vi "Stitch bottom tier.vi"(4 "Bottom tier Stitched Image":T1(plugin-control), 6 "Initial frame":bool, 8 "error in (no error)":errorcluster, 10 "Ctrl refs":T2, 11 "Input stitched image":T1) -> (0 "error out":errorcluster, 3 "Stitched Image":T1(plugin-control))   [LabVIEW 2013]
uses:
  <vilib>/vision/Image Controls.llb/IMAQ Image.ctl
  Typedefs/8-bit video export window ctrl refs.ctl
  Patch-Vol video generator/Typedefs/Bright-Contr-Gamma cluster.ctl
  Typedefs/Speed graph behaviour enum.ctl
  <vilib>/vision/NI_Vision_Development_Module.lvlib
panel:
  in  "AVI File Path":path=path "F:/Recovered data 03-24-2015 at 11_16_03/NTFS 1/LostFiles1/TimeLapse 03_10_2014 17-26-28 zoom1_50ns_MF_export/Green Channel 1.avi"
  out "Input stitched image":T1(plugin-control)
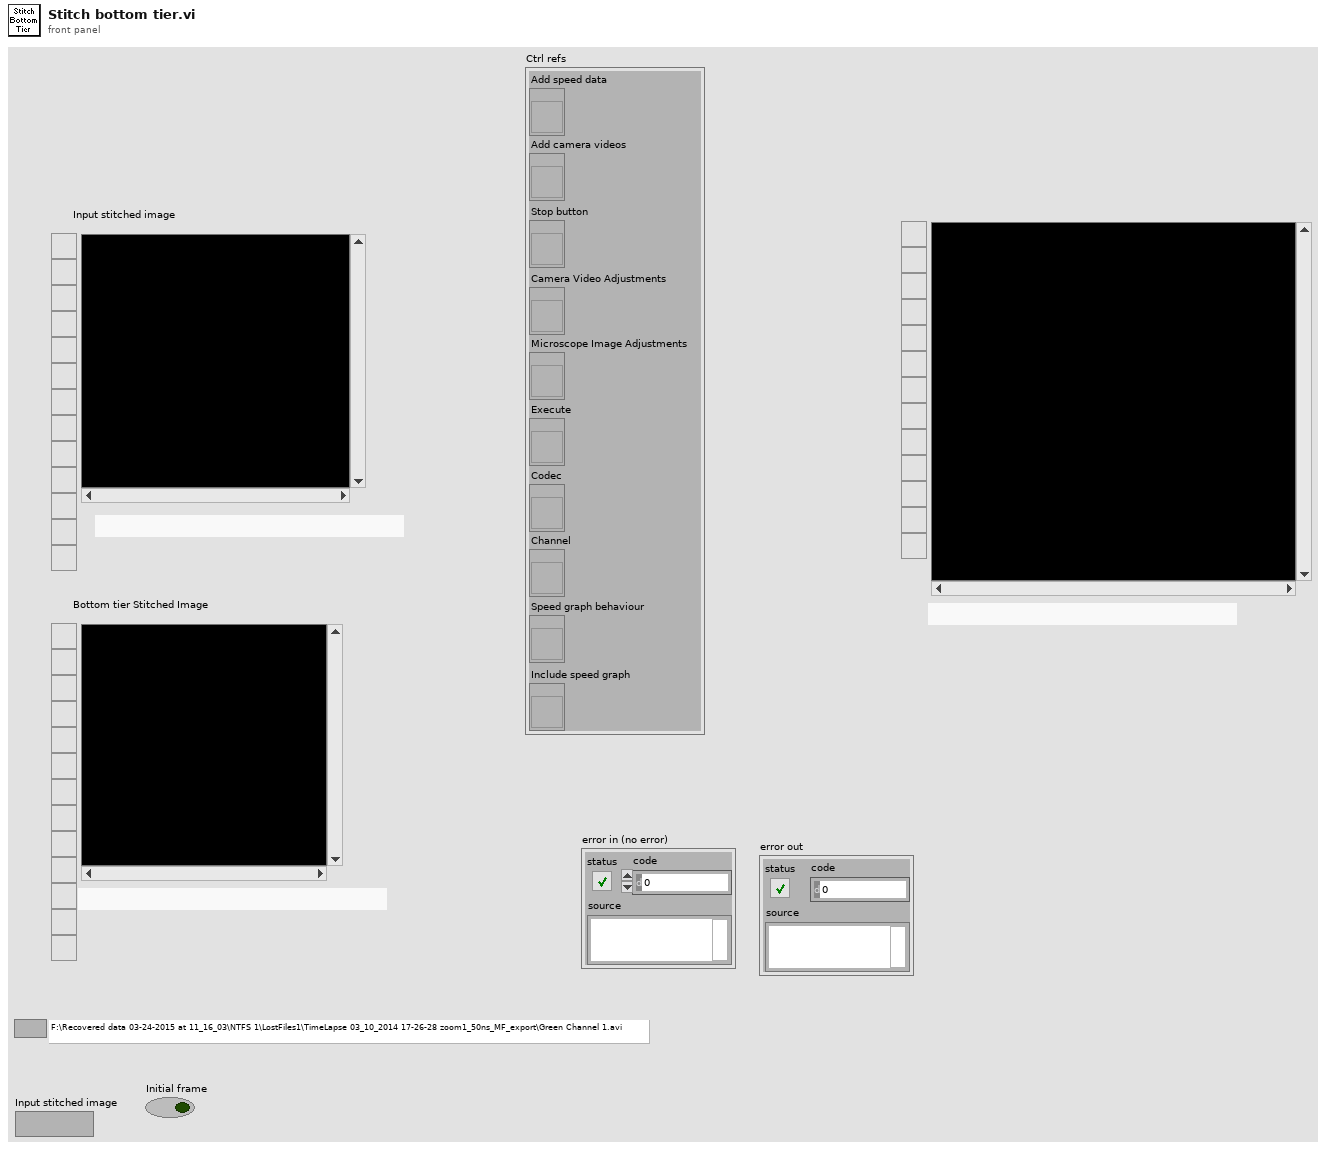
[diagram p1: front panel]
types:
  T1 = typedef "IMAQ Image.ctl" = refnum<image>
  T2 = typedef "8-bit video export window ctrl refs.ctl" = cluster{"Add speed data":refnum<vi>, "Add camera videos":refnum<vi>, "Stop button":refnum<vi>, "Camera Video Adjustments":refnum<vi>, "Microscope Image Adjustments":refnum<vi>, "Execute":refnum<vi>, "Codec":refnum<vi>, "Channel":refnum<vi>, "Speed graph behaviour":refnum<vi>, "Include speed graph":refnum<vi>}
  T3 = typedef "Image Type" = u32
  T4 = typedef "IMAQ AVI2 Refnum.ctl" = refnum<k20>
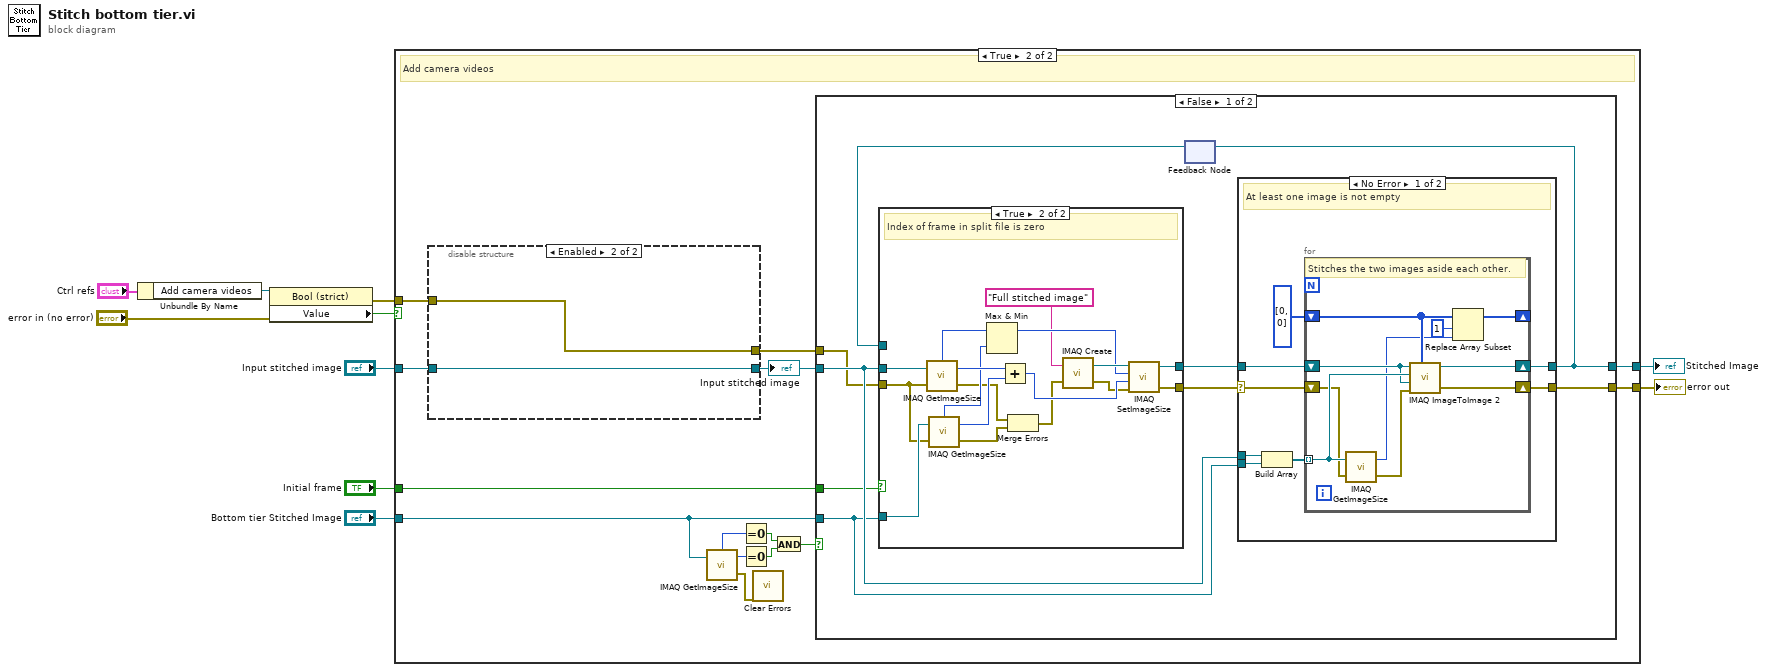
[diagram p0: block diagram]
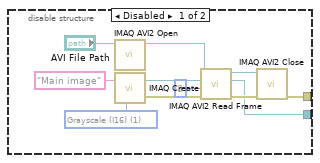
[diagram p6: hidden frame]
diagram:
  n1 = Unbundle By Name("Ctrl refs") -> ("Add camera videos"=w8:refnum<vi>)
  n2 = property class="Bool (strict)"(reference=w8, error in="error in (no error)") -> (error out=w4:errorcluster, "Value"=w6:bool)  [unwired: 1 out]
  n3 = case shown="True" w6 {
    tunnel: [w12 w24] -> w10
    tunnel: [w11 w25] -> w9
    tunnel: "Input stitched image" -> [w12 w26]
    tunnel: w4 -> [w11 w14]
    tunnel: "Initial frame" -> [_ w21]
    tunnel: "Bottom tier Stitched Image" -> [_ w20]
    frame False {
    }
    frame True {
      # "Add camera videos"
      n4 = disable-structure shown="Enabled" {
        disable-tunnel: [w78 w89] -> w23
        disable-tunnel: [w77 w88] -> w22
        disable-tunnel: w26 -> [_ w89]
        disable-tunnel: w14 -> [_ w88]
        frame Disabled {
          w85 = T3 1 items=["Grayscale (U8)", "Grayscale (I16)", "Grayscale (SGL)", "Complex (CSG)", "RGB (U32)", "HSL (U32)", "RGB (U64)", "Grayscale (U16)"] ("Image Type")
          n5 = call "IMAQ AVI2 Open"("AVI File Path"="AVI File Path") -> ("AVI Refnum"=w87:T4)  [unwired: 9 in, 1 out]
          n6 = call "IMAQ Create"("Image Name"="Main image", "Image Type"=w85) -> ("New Image"=w83:T1, "error out"=w82:errorcluster)  [unwired: 3 in]
          n7 = call "IMAQ AVI2 Read Frame"("error in (no error)"=w82, "Frame Number"=u32 3, "Image"=w83, "AVI Refnum"=w87) -> ("error out"=w81:errorcluster, "Image Out"=w78:T1, "AVI Refnum (duplicate)"=w86:T4)  [unwired: 5 in]
          n8 = call "IMAQ AVI2 Close"("error in (no error)"=w81, "AVI Refnum"=w86) -> ("error out"=w77:errorcluster)  [unwired: 9 in]
        }
        frame Enabled {
        }
      }
      "Input stitched image" <- w23
      n9 = call "IMAQ GetImageSize"("Image"=w20) -> ("Y Resolution"=w19:i32, "X Resolution"=w18:i32, "error out"=w13:errorcluster)  [unwired: 3 in]
      n10 = Equal To 0?(x=w18) -> (x = 0?=w17:bool)
      n11 = Equal To 0?(x=w19) -> (x = 0?=w16:bool)
      n12 = call <vilib>:"Clear Errors.vi"("error in (no error)"=w13) -> ()  [unwired: 6 in, 1 out]
      n13 = And(x=w17, y=w16) -> (x .and. y?=w15:bool)
      n14 = case shown="False" w15 {
        tunnel: [w35 w75] -> w25
        tunnel: [w34 w76] -> w24
        tunnel: w23 -> [w31 w76]
        tunnel: w22 -> [w30 w75]
        tunnel: w21 -> [w29 _]
        tunnel: w20 -> [w27 _]
        frame False {
          n15 = feedback #1() -> (w28:T1)  [unwired: 1 in]
          n16 = case shown="True" w29 {
            tunnel: w31 -> [_ w74]
            tunnel: w30 -> [w57 w64]
            tunnel: w27 -> [_ w73]
            tunnel: [w57 w59] -> w32
            tunnel: [w56 w58] -> w33
            tunnel: w28 -> [w56 _]
            frame False {
            }
            frame True {
              # "Index of frame in split file is zero"
              n17 = call "IMAQ GetImageSize"("Image"=w74, "error in (no error)"=w64) -> ("Y Resolution"=w70:i32, "X Resolution"=w68:i32, "error out"=w63:errorcluster)  [unwired: 2 in]
              n18 = call "IMAQ GetImageSize"("Image"=w73, "error in (no error)"=w64) -> ("Y Resolution"=w71:i32, "X Resolution"=w69:i32, "error out"=w62:errorcluster)  [unwired: 2 in]
              n19 = Max & Min(x=w68, y=w69) -> (max(x,y)=w67:i32)  [unwired: 1 out]
              n20 = Add(x=w70, y=w71) -> (x+y=w66:i32)
              n21 = Merge Errors(w63, w62) -> (w61:errorcluster)
              n22 = call "IMAQ Create"("Image Name"="Full stitched image", "error in (no error)"=w61) -> ("New Image"=w72:T1, "error out"=w65:errorcluster)  [unwired: 2 in, 1 out]
              n23 = call "IMAQ SetImageSize"("error in (no error)"=w65, "Y Resolution"=w66, "X Resolution"=w67, "Image"=w72) -> ("error out"=w59:errorcluster, "Image Out"=w58:T1)  [unwired: 1 out]
            }
          }
          n24 = case shown="No Error" w32 {
            selector: w32 -> [w36 w55]
            tunnel: w33 -> [w37 w54]
            tunnel: w31 -> [w41 _]
            tunnel: w27 -> [w40 _]
            tunnel: [w39 w55] -> w35
            tunnel: [w38 w54] -> w34
            frame No Error {
              # "At least one image is not empty"
              n25 = Build Array(w41, w40) -> (w42:T1[])
              n26 = for {
                tunnel: w42 -> [w53] mode=indexing
                shift-right: [w52] -> _
                shift-left: i32[] [0, 0] -> [w51]
                shift-right: [w49] -> w38
                shift-left: w37 -> [w47]
                shift-right: [w45] -> w39
                shift-left: w36 -> [w46]
                # "Stitches the two images aside each other."
                n27 = call "IMAQ GetImageSize"("Image"=w53, "error in (no error)"=w46) -> ("Y Resolution"=w44:i32, "error out"=w48:errorcluster)  [unwired: 3 out]
                n28 = call "IMAQ ImageToImage 2"("Offset Left/Top"=w51, "error in (no error)"=w48, "Image Dst"=w47, "Image Src (Small)"=w53, "Image Src (Large)"=w47) -> ("error out"=w45:errorcluster, "Image Dst Out"=w49:T1)  [unwired: 1 in, 4 out]
                n29 = Replace Array Subset(array=w51, new element=w44, index=1) -> (w52:i32[])
              }
            }
            frame Error {
              # "Both images are empty"
            }
          }
          n30 = feedback-in #1(w34) -> ()
        }
        frame True {
          # "Empty bottom tier image"
        }
      }
    }
  }
  "Stitched Image" <- w10
  "error out" <- w9
